vi "SetAPSxRefCurveVal.vi"(0 "hASIC":i32, 1 "LeftX":dbl, 2 "LeftY":dbl, 3 "RightX":dbl, 4 "RightY":dbl, 5 "error in (no error)":errorcluster caption="错误输入（无错误）", 6 "LowerLimit":dbl, 7 "iNumNPoint":i32, 8 "UpperLimit":dbl, 9 "pNPointX":dbl, 10 "yScale":dbl, 11 "pNPointY":dbl) -> (14 "hASIC out":i32, 15 "Message":string, 19 "error out":errorcluster caption="错误输出")   [LabVIEW 2020]
doc: "该模板用于创建子VI。"
uses:
  APSx.dll/APSx.dll
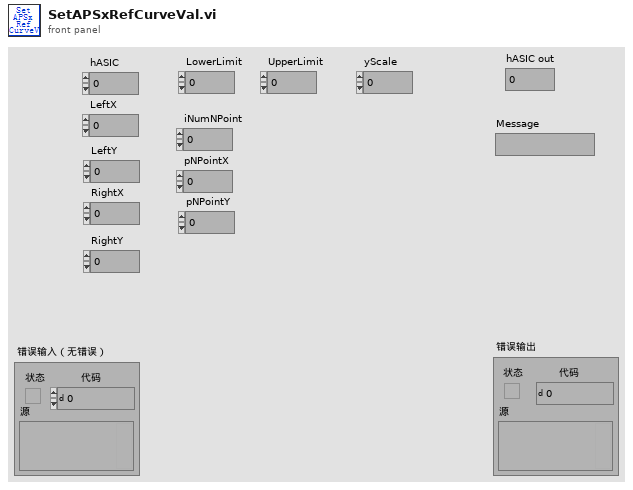
[diagram p1: front panel]
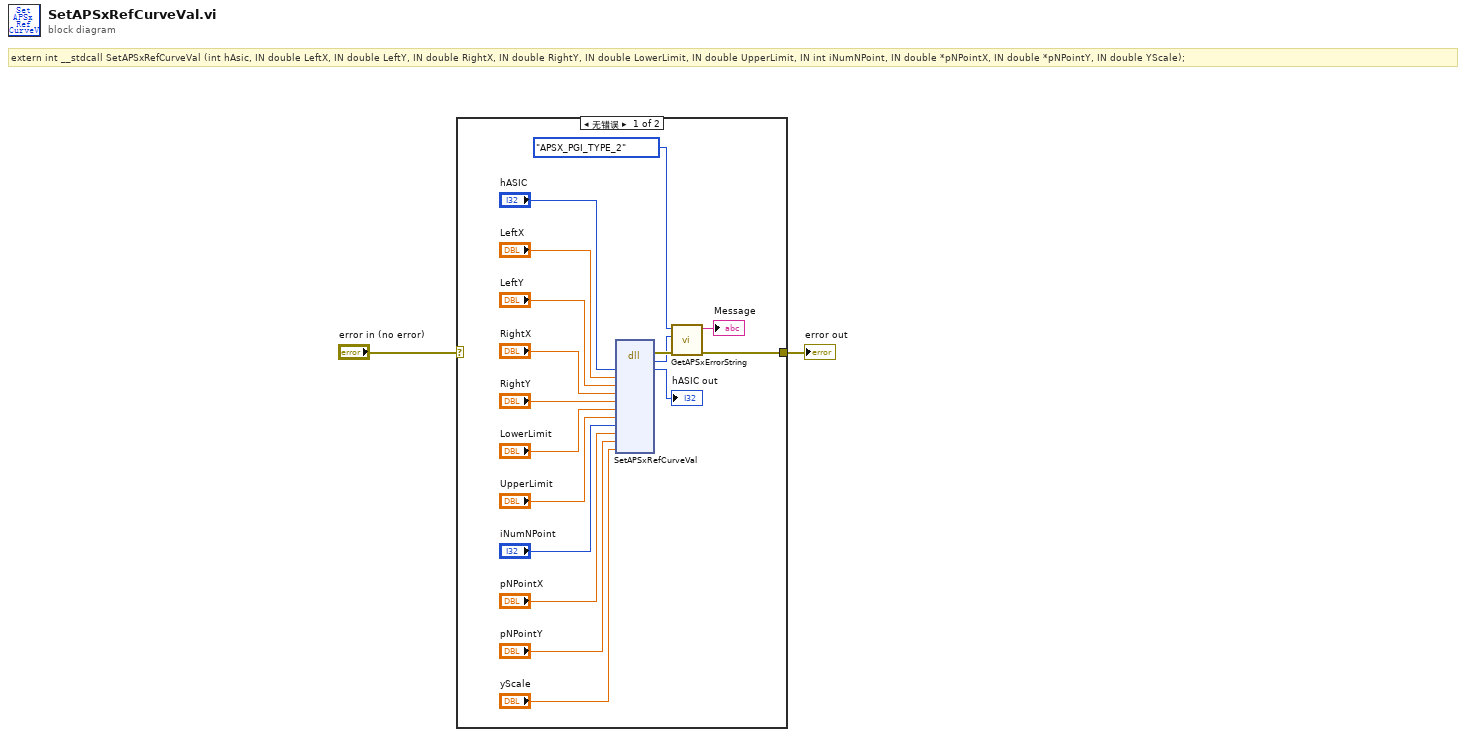
[diagram p0: block diagram]
diagram:
  # "extern int __stdcall SetAPSxRefCurveVal (int hAsic, IN double LeftX, IN double LeftY, IN double RightX, IN double RightY, IN double LowerLimit, IN double UpperLimit, IN int iNumNPoint, IN double *pNPointX, IN double *pNPointY, IN double YScale);"
  n1 = case shown="无错误" "error in (no error)" {
    selector: "error in (no error)" -> [_ w20]
    tunnel: [w9 w20] -> w1
    frame No Error {
      n2 = dll-call lib="PTH2iabs CUsersFengDesktop传感器对中台传感器对中台labviewSourcesAPSx.dllAPSx.dll" fn="SetAPSxRefCurveVal"("hASIC"="hASIC", "LeftX"="LeftX", "LeftY"="LeftY", "RightX"="RightX", "RightY"="RightY", "LowerLimit"="LowerLimit", "UpperLimit"="UpperLimit", "iNumNPoint"="iNumNPoint", "pNPointX"="pNPointX", "pNPointY"="pNPointY", "yScale"="yScale") -> (error out=w10:errorcluster, "Code"=w8:i32, "hASIC"=→"hASIC out":i32)  [unwired: 13 in, 1 out]
      n3 = call "GetAPSxErrorString.vi"("error in (no error)"=w10, "ErrorCode"=w8, "PGIType"=enum16{"APSX_PGI_TYPE_1", "APSX_PGI_TYPE_2"}."APSX_PGI_TYPE_2") -> ("error out"=w9:errorcluster, "Message"=→"Message":string)  [unwired: 7 in]
    }
    frame Error {
    }
  }
  "error out" <- w1
